vi "risingEdge.vi"(1 "In":bool) -> (0 "out":bool)   [LabVIEW 2014]
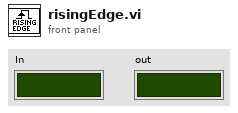
[diagram p1: front panel]
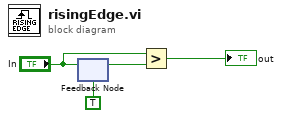
[diagram p0: block diagram]
diagram:
  n1 = feedback-in #1("In") -> ()
  n2 = feedback #1(TRUE ("In")) -> (w4:bool)
  n3 = Greater?(x="In", y=w4) -> (0:→"out":bool)
